vi "Mutex Lock.vi"(8 "error in (no error)":errorcluster, 11 "Mutex in":T1) -> (0 "error out":errorcluster, 3 "Mutex out":T1)   [LabVIEW 2013, in "Linux RT IPC.POSIX Threads.lvlib" / "Mutex.lvclass"]
doc: "Calls pthread_mutex_lock() on the pthread mutex object encapsulated by Mutex.\n\nThis VI attempts to lock the provided mutex. If already locked, this VI will wait indefinitely to try and lock the mutex. If not locked, the mutex will be locked and this VI will return immediately.\n\nRefer to online POSIX documentation for more information."
uses:
  Mutex.lvclass
  Controls/reference.ctl
  POSIX Thread Object/POSIX Thread Object.lvclass/POSIX Thread Object.ctl
  POSIX Thread Object/Private VIs/libpthread path.vi
  POSIX Thread Object/Private VIs/get pthread error.vi
  POSIX Thread Object/POSIX Thread Object.lvclass
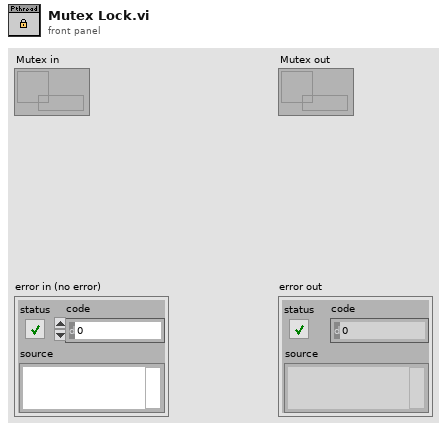
[diagram p1: front panel]
types:
  T1 = typedef "Linux RT IPC.POSIX Threads.lvlib/Mutex.lvclass/reference.ctl" = refnum<data-value>
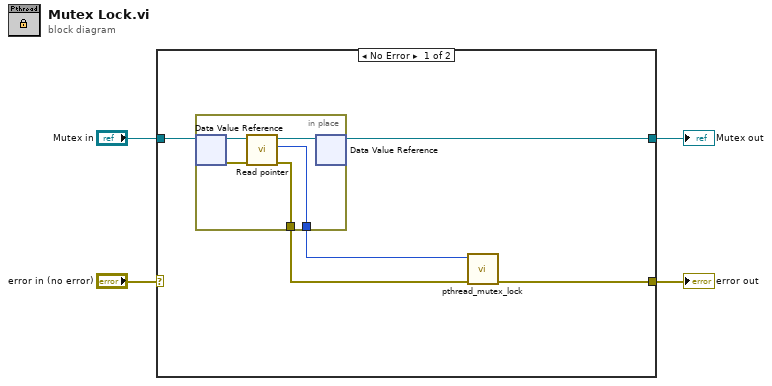
[diagram p0: block diagram]
diagram:
  n1 = case shown="No Error" "error in (no error)" {
    selector: "error in (no error)" -> [_ w16]
    tunnel: [w9 w16] -> w3
    tunnel: "Mutex in" -> [w8 w15]
    tunnel: [w5 w15] -> w1
    frame No Error {
      n2 = in-place {
        in-place-border: [w11] -> w7
        in-place-border: [w10] -> w6
        n3 = in-place-dvr #1(w8) -> (w14:refnum<class "Mutex.lvclass">, w12:errorcluster)
        n4 = call "Read pointer.vi"("error in (no error)"=w12, "POSIX Thread Object in"=w14) -> ("error out"=w11:errorcluster, "pointer"=w10:u64, "POSIX Thread Object out"=w13:refnum<class "Mutex.lvclass">)  [unwired: 7 in]
        n5 = in-place-dvr #1(w13) -> (w5:T1)  [unwired: 1 out]
      }
      n6 = call "pthread_mutex_lock.vi"("error in (no error)"=w7, "mutex ptr in"=w6) -> ("error out"=w9:errorcluster)  [unwired: 8 in, 1 out]
    }
    frame Error {
    }
  }
  "Mutex out" <- w1
  "error out" <- w3
